vi "SET_Glyph.vi"(8 "error in":errorcluster, 10 "Coordinates":T5, 11 "Data in":T1={"Class"={"Ants"=refnum, "Layer"=refnum, "Templates"=refnum, "Icon"=refnum, "Glyph"=refnum, "Settings"=refnum, "Tools"=refnum}, "Ref"={"Add Layer"=refnum, "Remove Layer"=refnum, "Line Text"=[], "Body Text Spec"=refnum, "DNL_Font"=refnum, "glyph path str"=refnum, "templates path str"=refnum, "Arrow Up"=refnum, "Arrow Down"=refnum, "IE VI Ref"=refnum, "Glyphs tree"=refnum, "Templates tree"=refnum, "Layer Icon Text"=refnum, "Layer Template"=refnum, "Body Text"=refnum, "Search Templates"=refnum, "TextMarker"=refnum, "Tab Control"=refnum, "Search Glyphs"=refnum, "Line Color"=refnum, "DNL_Glyphs []"=refnum, "Fill Color"=refnum, "Tools"=refnum, "Icon"=refnum, "Preview"=refnum, "Ants"=refnum, "Terminals"=refnum, "menu reference"=refnum, "LayerNames"=[], "GlyphLoadAnimation"=refnum, "TemplateLoadAnimation"=refnum, "refreshGlyphs"=refnum, "refreshTemplates"=refnum}, "Support"={"AntsRect"={"left"=0, "top"=0, "right"=0, "bottom"=0}, "Mouse Move Coords"={"Horizontal"=0, "Vertical"=0}, "Mouse Down Coords"={"Horizontal"=0, "Vertical"=0}, "Temp Coord"={"Horizontal"=0, "Vertical"=0}, "Action"=enum."Default", "Edge Color"=4914962, "Fill Color"=16860, "Mouse Down?"=FALSE, "Draft Mode?"=FALSE, "Temp Icon"=bytes[3102], "CTRL Pressed"=FALSE, "Move Selection?"=FALSE, "AntsRect Orig"={"left"=0, "top"=0, "right"=0, "bottom"=0}, "Text"="", "TM Set?"=FALSE, "Mouse inside icon?"=FALSE, "Tool (old value)"=0, "Pencil Move Color"=0, "Swap Colors?"=FALSE, "Shift pressed?"=FALSE}}) -> (0 "error out":errorcluster, 1 "All Layers":refnum<class "Layer.lvclass">[](array[class]), 3 "Data out":T1={"Class"={"Ants"=refnum, "Layer"=refnum, "Templates"=refnum, "Icon"=refnum, "Glyph"=refnum, "Settings"=refnum, "Tools"=refnum}, "Ref"={"Add Layer"=refnum, "Remove Layer"=refnum, "Line Text"=[], "Body Text Spec"=refnum, "DNL_Font"=refnum, "glyph path str"=refnum, "templates path str"=refnum, "Arrow Up"=refnum, "Arrow Down"=refnum, "IE VI Ref"=refnum, "Glyphs tree"=refnum, "Templates tree"=refnum, "Layer Icon Text"=refnum, "Layer Template"=refnum, "Body Text"=refnum, "Search Templates"=refnum, "TextMarker"=refnum, "Tab Control"=refnum, "Search Glyphs"=refnum, "Line Color"=refnum, "DNL_Glyphs []"=refnum, "Fill Color"=refnum, "Tools"=refnum, "Icon"=refnum, "Preview"=refnum, "Ants"=refnum, "Terminals"=refnum, "menu reference"=refnum, "LayerNames"=[], "GlyphLoadAnimation"=refnum, "TemplateLoadAnimation"=refnum, "refreshGlyphs"=refnum, "refreshTemplates"=refnum}, "Support"={"AntsRect"={"left"=0, "top"=0, "right"=0, "bottom"=0}, "Mouse Move Coords"={"Horizontal"=0, "Vertical"=0}, "Mouse Down Coords"={"Horizontal"=0, "Vertical"=0}, "Temp Coord"={"Horizontal"=0, "Vertical"=0}, "Action"=enum."Default", "Edge Color"=4914962, "Fill Color"=16860, "Mouse Down?"=FALSE, "Draft Mode?"=FALSE, "Temp Icon"=bytes[3102], "CTRL Pressed"=FALSE, "Move Selection?"=FALSE, "AntsRect Orig"={"left"=0, "top"=0, "right"=0, "bottom"=0}, "Text"="", "TM Set?"=FALSE, "Mouse inside icon?"=FALSE, "Tool (old value)"=0, "Pencil Move Color"=0, "Swap Colors?"=FALSE, "Shift pressed?"=FALSE}})   [LabVIEW 2020]
uses:
  vi.lib/LabVIEW Icon API/lv_icon/Classes/Icon/Icon.lvclass
  vi.lib/LabVIEW Icon API/lv_icon/Classes/Layer/Layer.lvclass
  vi.lib/LabVIEW Icon API/lv_icon/Controls/LayerType.ctl
  Class/Icon Library/Glyph.lvclass
  Class/FakedArray/FakedArray.lvclass
  <vilib>/Utility/miscctls.llb/LVPoint32TypeDef.ctl
  Controls/SupportClass_Action.ctl
  vi.lib/LabVIEW Icon API/lv_icon/Controls/IEColor.ctl
  Controls/SupportClass.ctl
  Controls/References Cluster.ctl
  vi.lib/LabVIEW Icon API/lv_icon/lv_icon.lvlib
  Class/Tools/Tools Paint.lvclass
  Class/Settings/Settings.lvclass
  Class/Ants/Ants.lvclass
  Controls/IE Classes.ctl
  Controls/Global Data.ctl
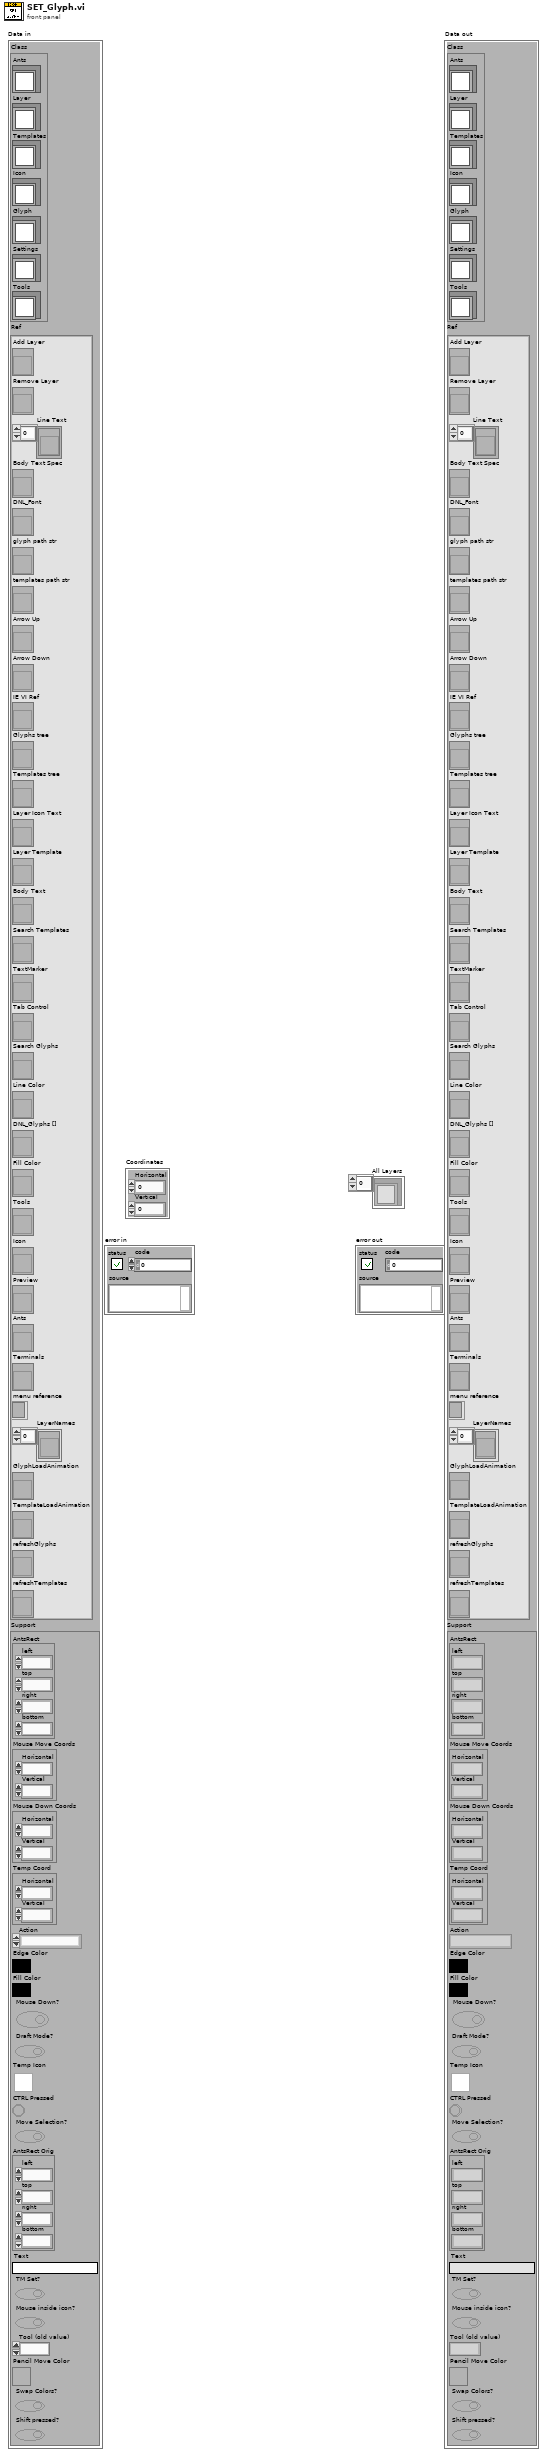
[diagram p1: front panel]
types:
  T1 = typedef "lv_icon.lvlib/Global Data.ctl" = cluster{"Class":T2, "Ref":T3, "Support":T4}
  T2 = typedef "IE Classes.ctl" = cluster{"Ants":refnum<class "Ants.lvclass">, "Layer":refnum<class "FakedArray.lvclass">, "Templates":refnum<class "FakedArray.lvclass">, "Icon":refnum<class "Icon.lvclass">, "Glyph":refnum<class "Glyph.lvclass">, "Settings":refnum<class "Settings.lvclass">, "Tools":refnum<class "Tools Paint.lvclass">}
  T3 = typedef "lv_icon.lvlib/References Cluster.ctl" = cluster{"Add Layer":refnum<vi>, "Remove Layer":refnum<vi>, "Line Text":refnum<vi>[], "Body Text Spec":refnum<vi>, "DNL_Font":refnum<vi>, "glyph path str":refnum<vi>, "templates path str":refnum<vi>, "Arrow Up":refnum<vi>, "Arrow Down":refnum<vi>, "IE VI Ref":refnum<vi>, "Glyphs tree":refnum<vi>, "Templates tree":refnum<vi>, "Layer Icon Text":refnum<vi>, "Layer Template":refnum<vi>, "Body Text":refnum<vi>, "Search Templates":refnum<vi>, "TextMarker":refnum<vi>, "Tab Control":refnum<vi>, "Search Glyphs":refnum<vi>, "Line Color":refnum<vi>, "DNL_Glyphs []":refnum<vi>, "Fill Color":refnum<vi>, "Tools":refnum<vi>, "Icon":refnum<vi>, "Preview":refnum<vi>, "Ants":refnum<vi>, "Terminals":refnum<vi>, "menu reference":refnum<k9>, "LayerNames":refnum<vi>[], "GlyphLoadAnimation":refnum<vi>, "TemplateLoadAnimation":refnum<vi>, "refreshGlyphs":refnum<vi>, "refreshTemplates":refnum<vi>}
  T4 = typedef "SupportClass.ctl" = cluster{"AntsRect":cluster{"left":i16, "top":i16, "right":i16, "bottom":i16}, "Mouse Move Coords":T5, "Mouse Down Coords":T5, "Temp Coord":T5, "Action":T6, "Edge Color":T7, "Fill Color":T7, "Mouse Down?":bool, "Draft Mode?":bool, "Temp Icon":picture, "CTRL Pressed":bool, "Move Selection?":bool, "AntsRect Orig":cluster{"left":i16, "top":i16, "right":i16, "bottom":i16}, "Text":string, "TM Set?":bool, "Mouse inside icon?":bool, "Tool (old value)":u32, "Pencil Move Color":u32, "Swap Colors?":bool, "Shift pressed?":bool}
  T5 = typedef "LVPoint32TypeDef.ctl" = cluster{"Horizontal":i32, "Vertical":i32}
  T6 = typedef "SupportClass_Action.ctl" = enum16{"Default", "Move Selection", "Glyph Library", "Tool"}
  T7 = typedef "IEColor.ctl" = u32
  T8 = typedef "LayerType.ctl" = enum16{"Graphic", "Text", "Tool", "Graphic Drop"}
  T9 = typedef "Graphic.ctl" = cluster{"Rectangle":cluster{"left":i16, "top":i16, "right":i16, "bottom":i16}, "Path":path, "Image":picture, "Filter":string, "FileName":string}
  T10 = typedef "lv_icon.lvlib/INI Data.ctl" = cluster{"Show Terminals?":bool, "Text":cluster{"Font":T11, "Alignment":T12, "Size":T13}, "3rd party Templates":cluster{"Store 3rd party Templates?":bool, "Folder Name":string}, "Merge user layers on commit":bool, "Body Text":T14, "Fill Color":T7, "Edge Color":T7, "Tab":u16, "Tool":T15, "Disable Layers?":bool}
  T11 = typedef "Font.ctl" = string
  T12 = typedef "Alignment.ctl" = u16
  T13 = typedef "Font Size.ctl" = u8
  T14 = typedef "BodyText.ctl" = cluster{"Line 1 text":string, "Line 2 text":string, "Line 3 text":string, "Line 4 text":string, "Line 1 color":u32, "Line 2 color":u32, "Line 3 color":u32, "Line 4 color":u32, "Body Text Spec":cluster{"Font":T11, "Alignment":T12, "Size":u8}, "Center text vertically":bool, "Capitalize Text":bool}
  T15 = typedef "Tools.ctl" = enum32{"Pencil", "Line", "Dropper", "Fill", "Rectangle", "Filled Rectangle", "Ellipse", "Filled Ellipse", "Eraser", "Text", "Select", "Move"}
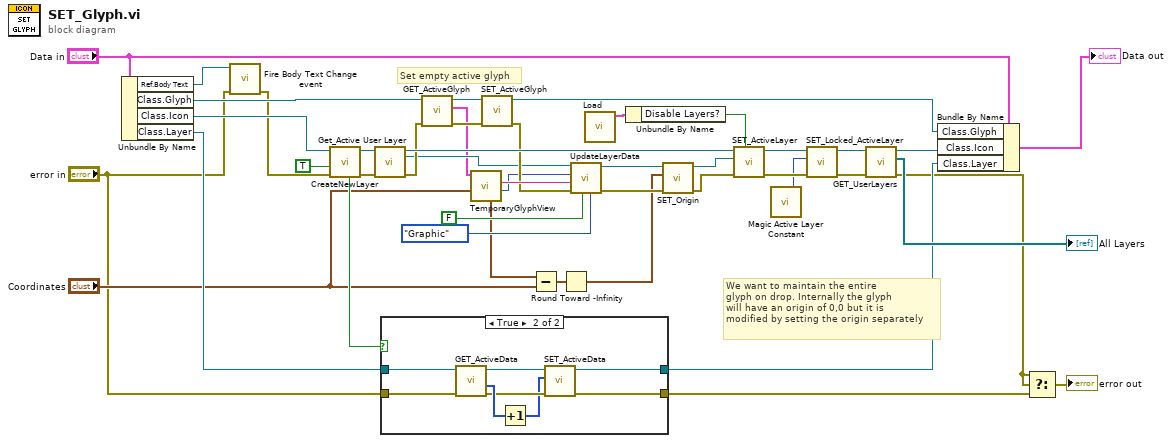
[diagram p0: block diagram]
diagram:
  # "We want to maintain the entire\nglyph on drop. Internally the glyph\nwill have an origin of 0,0 but it is\nmodified by setting the origin separately"
  # "Set empty active glyph"
  n1 = Unbundle By Name("Data in") -> ("Ref.Body Text"=w5:refnum<vi>, "Class.Glyph"=w25:refnum<class "Glyph.lvclass">, "Class.Icon"=w24:refnum<class "Icon.lvclass">, "Class.Layer"=w20:refnum<class "FakedArray.lvclass">)
  n2 = call "Fire Body Text Change event.vi"("error in"="error in", "Ref.Body Text"=w5) -> ("error out"=w3:errorcluster)  [unwired: 2 in, 7 out]
  n3 = call "CreateNewLayer.vi"("error in"=w3, "Force New Layer?"=TRUE, "Icon.lvclass"=w24) -> ("error out"=w36:errorcluster, "Icon.lvclass out"=w35:refnum<class "Icon.lvclass">, "Layer added?"=w29:bool)  [unwired: 2 in, 4 out]
  n4 = call-dynamic "Get_Active User Layer.vi"("error in (no error)"=w36, "Icon in"=w35) -> ("error out"=w38:errorcluster, "Layer.lvclass"=w37:refnum<class "Layer.lvclass">, "Icon out"=w42:refnum<class "Icon.lvclass">)  [unwired: 7 out]
  n5 = case shown="True" w29 {
    tunnel: "error in" -> [w47 w48]
    tunnel: [w47 w49] -> w28
    tunnel: w20 -> [w46 w51]
    tunnel: [w46 w50] -> w19
    frame False {
    }
    frame True {
      n6 = call-dynamic "GET_ActiveData.vi"("error in (no error)"=w48, "FakedArray in"=w51) -> ("error out"=w53:errorcluster, "Active Data []"=w54:i32[], "FakedArray out"=w55:refnum<class "FakedArray.lvclass">)  [unwired: 7 out]
      n7 = Increment(x=w54) -> (x+1=w52:i32[])
      n8 = call-dynamic "SET_ActiveData.vi"("error in (no error)"=w53, "Active Data"=w52, "FakedArray.lvclass in"=w55) -> ("error out"=w49:errorcluster, "FakedArray.lvclass out"=w50:refnum<class "FakedArray.lvclass">)  [unwired: 7 out]
    }
  }
  n9 = call-dynamic "GET_ActiveGlyph.vi"("error in (no error)"=w38, "Glyph.lvclass in"=w25) -> ("error out"=w40:errorcluster, "Path & Icon"=w18:T9, "Glyph.lvclass out"=w39:refnum<class "Glyph.lvclass">)  [unwired: 7 out]
  n10 = call "TemporaryGlyphView.vi"("Mouse Coords Pic"="Coordinates", "Path & Icon"=w18) -> ("origin"=w7:picture, "FileName"=w43:string, "Offset"=w8:cluster{"right":dbl, "bottom":dbl})  [unwired: 7 out]
  n11 = call-dynamic "SET_ActiveGlyph.vi"("error in (no error)"=w40, "Glyph in"=w39) -> ("error out"=w41:errorcluster, "Glyph out"=w21:refnum<class "Glyph.lvclass">)  [unwired: 1 in, 7 out]
  n12 = Subtract(x=w8, y="Coordinates") -> (x-y=w11:cluster{dbl, dbl})
  n13 = Round Toward -Infinity(1:w11) -> (0:w9:cluster{dbl, dbl})
  n14 = call "UpdateLayerData.vi"("Type"=LayerType."Graphic", "Overwrite?"=FALSE, "error in"=w41, "LayerName"=w43, "new picture"=w7, "Active Layer"=w37) -> ("error out"=w14:errorcluster, "Layer.lvclass out"=w15:refnum<class "Layer.lvclass">)  [unwired: 2 in, 2 out]
  n15 = call "Load.vi"() -> ("INI Data"=w2:T10)  [unwired: 3 in, 8 out]
  n16 = Unbundle By Name(w2) -> ("Disable Layers?"=w1:bool)
  n17 = call-dynamic "SET_Origin.vi"("error in"=w14, "Point32"=w9, "Layer.lvclass in"=w15) -> ("error out"=w12:errorcluster, "Layer.lvclass out"=w13:refnum<class "Layer.lvclass">)  [unwired: 7 out]
  n18 = call-dynamic "SET_ActiveLayer.vi"("Combine User Layers?"=w1, "error in (no error)"=w12, "Layer.lvclass"=w13, "Icon.lvclass in"=w42) -> ("error out"=w34:errorcluster, "Icon.lvclass out"=w31:refnum<class "Icon.lvclass">)  [unwired: 6 out]
  n19 = call "Magic Active Layer Constant.vi"() -> ("Magic Constant"=w26:i32)  [unwired: 19 out]
  n20 = call-dynamic "SET_Locked_ActiveLayer.vi"("error in (no error)"=w34, "Active Layer"=w26, "Icon.lvclass in"=w31) -> ("error out"=w33:errorcluster, "Icon.lvclass out"=w32:refnum<class "Icon.lvclass">)  [unwired: 1 in, 6 out]
  n21 = call-dynamic "GET_UserLayers.vi"("error in (no error)"=w33, "Icon.lvclass in"=w32) -> ("error out"=w17:errorcluster, "All Layers"=→"All Layers":refnum<class "Layer.lvclass">[], "Icon.lvclass out"=w22:refnum<class "Icon.lvclass">)  [unwired: 7 out]
  n22 = Bundle By Name(cluster="Data in", "Class.Glyph"=w21, "Class.Icon"=w22, "Class.Layer"=w19) -> (→"Data out":T1)
  n23 = Select(t=w17, s=w17, f=w28) -> (s? t:f=→"error out":errorcluster)
